vi "Initialize_DMM.vi"(8 "error in (no error)":errorcluster, 10 "DMM_Initialize":T1, 11 "DMM_Base in":refnum<class "DMM_Base.lvclass">) -> (0 "error out":errorcluster, 3 "DMM_Base out":refnum<class "DMM_Base.lvclass">)   [LabVIEW 2020, in "DMM_Base.lvclass"]
doc: "The API calls the initialization method of instrument connected to the pins given to <b>Reserve Sessions API</b>."
uses:
  DMM_Base.lvclass
  Typedef/DMM_Initialize.ctl
  <vilib>/MeasurementLink/MeasurementLink Session Management V1/Session Reservation/Initialize and Close Session Behavior.ctl
  DMM_Base.lvclass/DMM_Base.ctl
  <vilib>/MeasurementLink/MeasurementLink Session Management V1/Session Reservation/Session Reservation.lvclass
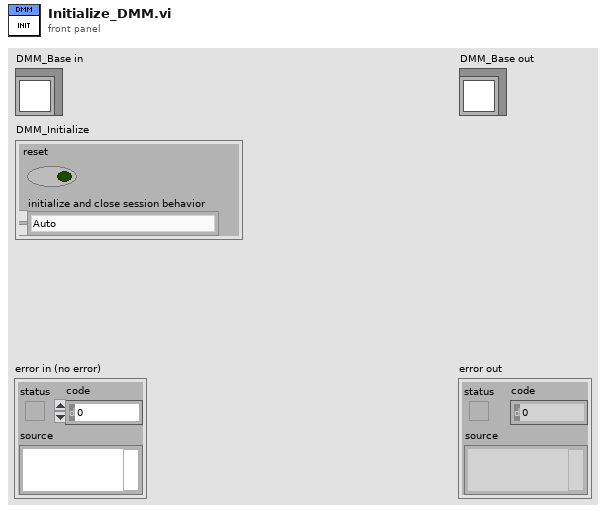
[diagram p1: front panel]
types:
  T1 = typedef "DMM_Base.lvclass/DMM_Initialize.ctl" = cluster{"initialize and close session behavior":T2, "reset":bool}
  T2 = typedef "MeasurementLink Session Management V1.lvlib/Session Reservation.lvclass/Initialize and Close Session Behavior.ctl" = enum16{"Auto", "Initialize and Close", "Attach and Detach", "Initialize and Detach", "Attach and Close"}
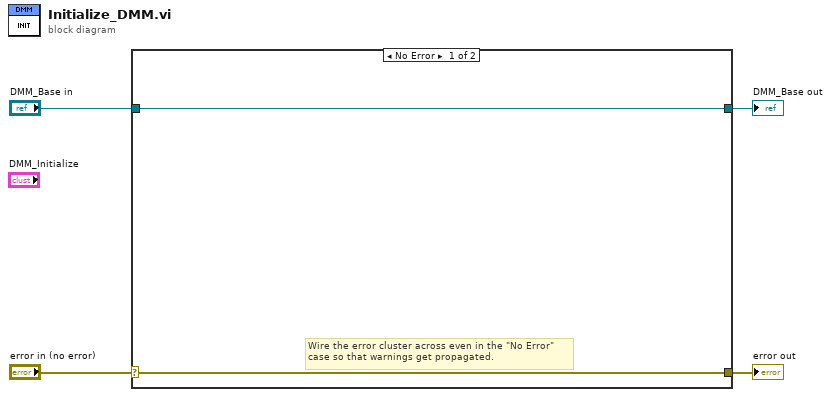
[diagram p0: block diagram]
diagram:
  n1 = case shown="No Error" "error in (no error)" {
    selector: "error in (no error)" -> [w5 w8]
    tunnel: [w5 w8] -> w3
    tunnel: [w6 w7] -> w1
    tunnel: "DMM_Base in" -> [w6 w7]
    frame No Error {
      # "Wire the error cluster across even in the \"No Error\"\ncase so that warnings get propagated."
    }
    frame Error {
    }
  }
  "error out" <- w3
  "DMM_Base out" <- w1
